vi "SLL DE Replace array subset.vi"(8 "error in (no error)":errorcluster, 9 "New element":string[](array[string]), 10 "Channel index":i32, 11 "Channel Name":string[][](array[string])) -> (0 "error out":errorcluster, 3 "Channel Name":string[][](array[string]))   [LabVIEW 2013]
doc: "Copyright © 2005, Soliton Technologies.\nAll rights reserved."
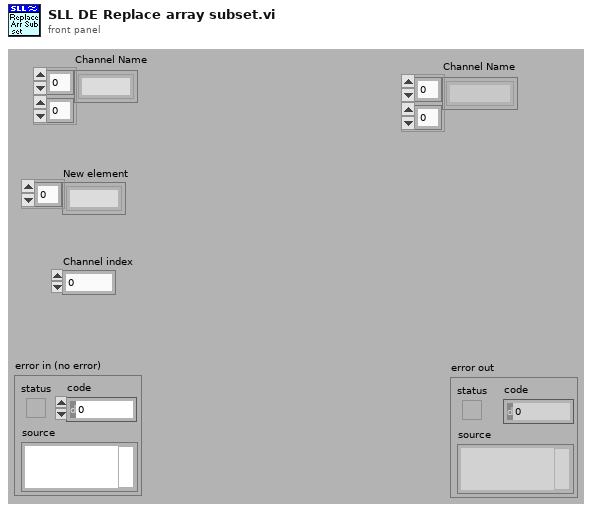
[diagram p1: front panel]
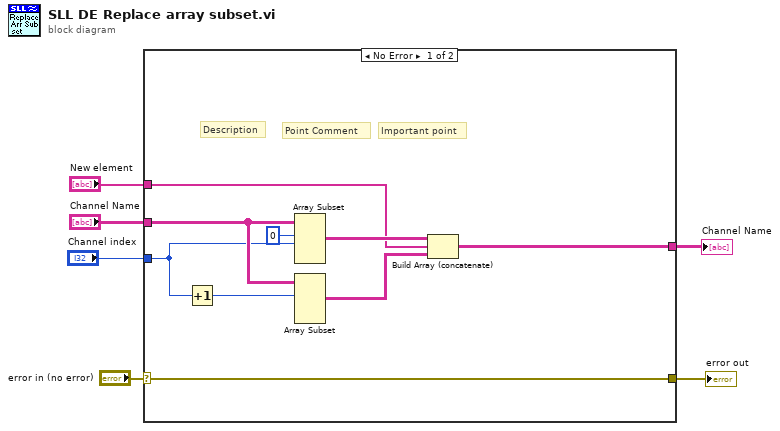
[diagram p0: block diagram]
diagram:
  n1 = case shown="No Error" "error in (no error)" {
    selector: "error in (no error)" -> [w15 w17]
    tunnel: [w15 w17] -> w5
    tunnel: "Channel Name" -> [w13 w16]
    tunnel: "Channel index" -> [w7 _]
    tunnel: "New element" -> [w10 _]
    tunnel: [w8 w16] -> w1
    frame No Error {
      # "Point Comment"
      # "Important point"
      # "Description"
      n2 = Increment(x=w7) -> (x+1=w12:i32)
      n3 = Array Subset(array=w13, index (row)=0 ("index"), length (row)=w7) -> (w11:string[][])  [unwired: 2 in]
      n4 = Array Subset(array=w13, index (row)=w12) -> (w9:string[][])  [unwired: 3 in]
      n5 = Build Array (concatenate)(w11, w10, w9) -> (w8:string[][])
    }
    frame Error {
    }
  }
  "error out" <- w5
  "Channel Name" <- w1
